vi "test Copy.vi"(8 "error in (no error)":errorcluster, 11 "TestCase in":refnum<class "Data Manipulation Tests.lvclass">) -> (0 "error out":errorcluster, 3 "TestCase out":refnum<class "Data Manipulation Tests.lvclass">)   [LabVIEW 2017, in "Pointer Tests.lvlib" / "Data Manipulation Tests.lvclass"]
uses:
  Data Manipulation Tests.lvclass
  Source/Classes/Pointer/Public/New/New (4B).vi
  Source/Classes/Pointer/Public/Write/Write (1D I32).vi
  <vilib>/addons/_JKI Toolkits/VI Tester/TestCase.llb/TestCase.lvclass
  Source/Classes/Pointer/Pointer.lvclass
  C:/Program Files (x86)/National Instruments/LabVIEW 2017/vi.lib/addons/_JKI Toolkits/VI Tester/TestCase.llb/TestCase.lvclass
panel:
  out "equal contents?":bool
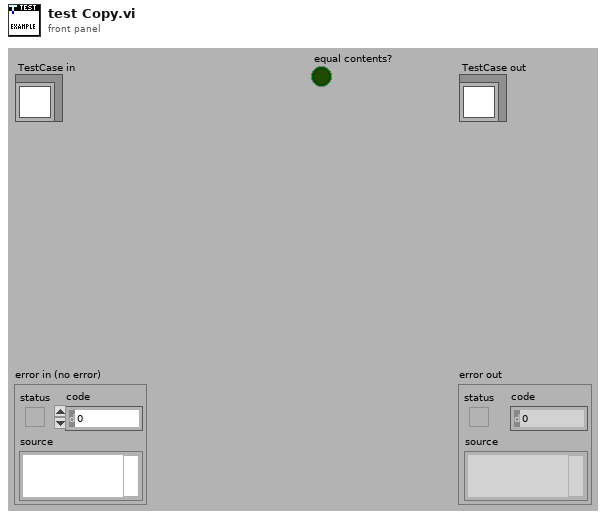
[diagram p1: front panel]
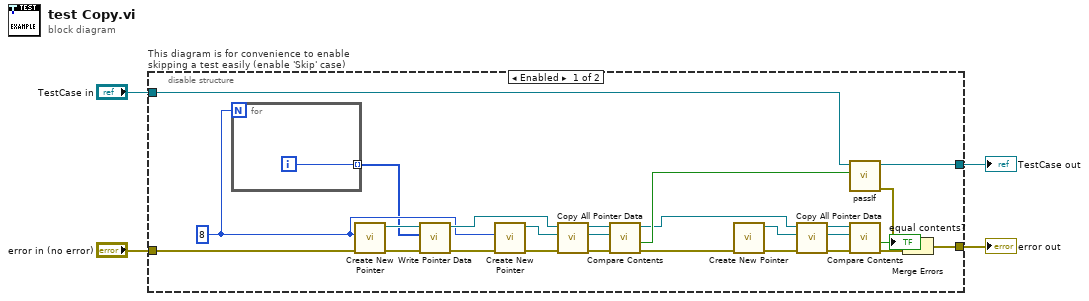
[diagram p0: block diagram]
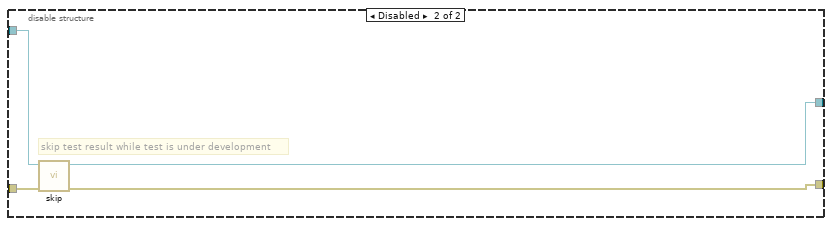
[diagram p2: hidden frame]
diagram:
  n1 = disable-structure "This diagram is for convenience to enable skipping a test easily (enable 'Skip' case)" shown="Enabled" {
    disable-tunnel: "TestCase in" -> [w22 w35]
    disable-tunnel: [w21 w33] -> w1
    disable-tunnel: [w15 w34] -> w3
    disable-tunnel: "error in (no error)" -> [w19 w32]
    frame Enabled {
      w28 = u64 8 ("count (1)")
      n2 = for {
        N: w28 -> [_]
        tunnel: [w31] -> w27 mode=indexing
        i -> [w31]
      }
      n3 = call-poly "Create New Pointer.vi"("error in (no error)"=w19, "count (1)"=w28) -> ("error out"=w18:errorcluster, "Pointer"=w30:refnum<class "Pointer.lvclass">)  [unwired: 8 in]
      n4 = call-poly "Write Pointer Data.vi"("error in (no error)"=w18, "buffer in"=w27, "Pointer in"=w30) -> ("error out"=w17:errorcluster, "Pointer out"=w29:refnum<class "Pointer.lvclass">)  [unwired: 5 in, 2 out]
      n5 = call-poly "Create New Pointer.vi"("error in (no error)"=w17, "count (1)"=w28) -> ("error out"=w16:errorcluster, "Pointer"=w26:refnum<class "Pointer.lvclass">)  [unwired: 8 in]
      n6 = call "Copy All Pointer Data.vi"("error in (no error)"=w16, "dst Pointer in"=w26, "src Pointer in"=w29) -> ("error out"=w13:errorcluster, "dst Pointer out"=w24:refnum<class "Pointer.lvclass">, "src Pointer out"=w25:refnum<class "Pointer.lvclass">)  [unwired: 6 in]
      n7 = call "Compare Contents.vi"("error in (no error)"=w13, "Pointer b in"=w24, "Pointer a in"=w25) -> ("error out"=w14:errorcluster, "equal contents?"=w20:bool, "Pointer a out"=w12:refnum<class "Pointer.lvclass">)  [unwired: 5 in, 1 out]
      n8 = call-poly "Create New Pointer.vi"("error in (no error)"=w14) -> ("error out"=w10:errorcluster, "Pointer"=w11:refnum<class "Pointer.lvclass">)  [unwired: 9 in]
      n9 = call "Copy All Pointer Data.vi"("error in (no error)"=w10, "dst Pointer in"=w11, "src Pointer in"=w12) -> ("error out"=w7:errorcluster, "dst Pointer out"=w8:refnum<class "Pointer.lvclass">, "src Pointer out"=w9:refnum<class "Pointer.lvclass">)  [unwired: 6 in]
      n10 = call-dynamic "passIf.vi"("pass"=w20, "TestCase in"=w22) -> ("error out"=w23:errorcluster, "TestCase out"=w21:refnum<class "Data Manipulation Tests.lvclass">)  [unwired: 8 in]
      n11 = call "Compare Contents.vi"("error in (no error)"=w7, "Pointer b in"=w8, "Pointer a in"=w9) -> ("error out"=w6:errorcluster, "equal contents?"=→"equal contents?":bool)  [unwired: 5 in, 2 out]
      n12 = Merge Errors(w23, w6) -> (w15:errorcluster)
    }
    frame Disabled {
      # "skip test result while test is under development"
      n13 = call <vilib>:"skip.vi"("error in (no error)"=w32, "TestCase in"=w35) -> ("error out"=w34:errorcluster, "TestCase out"=w33:refnum<class "Data Manipulation Tests.lvclass">)  [unwired: 8 in]
    }
  }
  "error out" <- w3
  "TestCase out" <- w1
